vi "DbFetchRecordThroughRecordNumber.vi"() -> ()   [LabVIEW 2019]
uses:
  <vilib>/addons/database/Recordset.llb/Rec Properties.ctl
  <vilib>/addons/database/Auxilliary.llb/DB Tools Cursor Type.ctl
  <vilib>/addons/database/Connection.llb/DB Tools Open Connec (String).vi
  <vilib>/addons/database/Connection.llb/Conn Execute.vi
  <vilib>/addons/database/Recordset.llb/Rec Get Recordset Properties (R).vi
  <vilib>/addons/database/Recordset.llb/Rec Move To Record N (R).vi
  <vilib>/addons/database/Recordset.llb/Rec Fetch String Data (R).vi
  <vilib>/addons/database/Recordset.llb/Rec Destroy - Connection.vi
  <vilib>/addons/database/NI_Database_API.lvlib
panel:
  out "Subject Name":string
  in  "Provide Index of Record":dbl
  in  "stop":bool
  in  "Get Records":bool
  out "Recordset Properties":T1
  in  "Table Name":string
  in  "Provide your ODBC server name":string
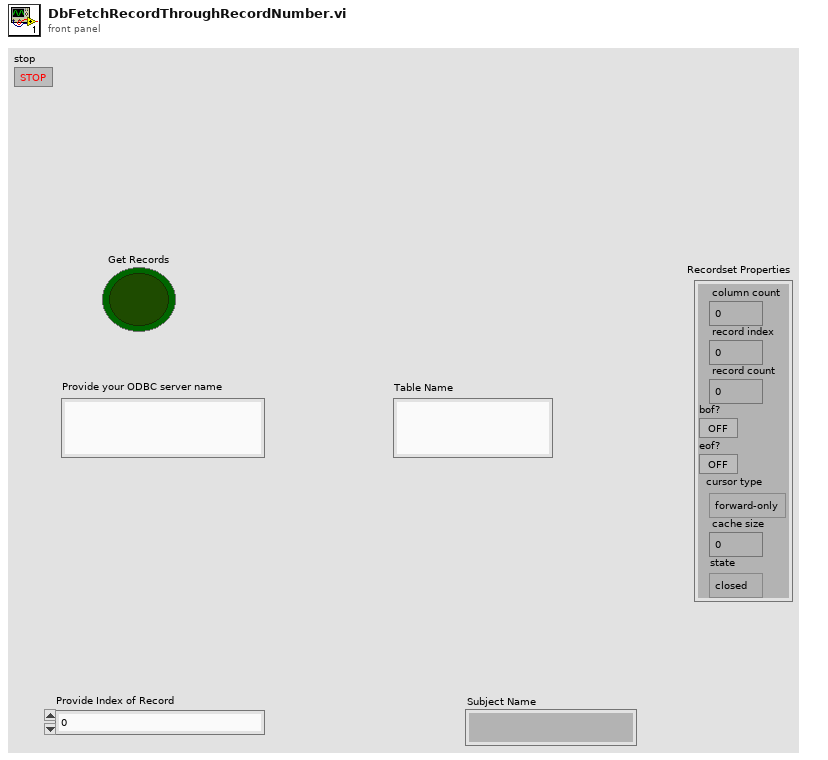
[diagram p1: front panel]
types:
  T1 = typedef "NI_Database_API.lvlib/Rec Properties.ctl" = cluster{"column count":i32, "record index":i32, "record count":i32, "bof?":bool, "eof?":bool, "cursor type":T2, "cache size":i32, "state":enum16{"closed", "open"}}
  T2 = typedef "NI_Database_API.lvlib/DB Tools Cursor Type.ctl" = enum16{"forward-only", "keyset", "dynamic", "static"}
  T3 = typedef "NI_Database_API.lvlib/Conn ObjectReference.ctl" = refnum<k1>
  T4 = typedef "NI_Database_API.lvlib/Rec ObjectReference.ctl" = refnum<k1>
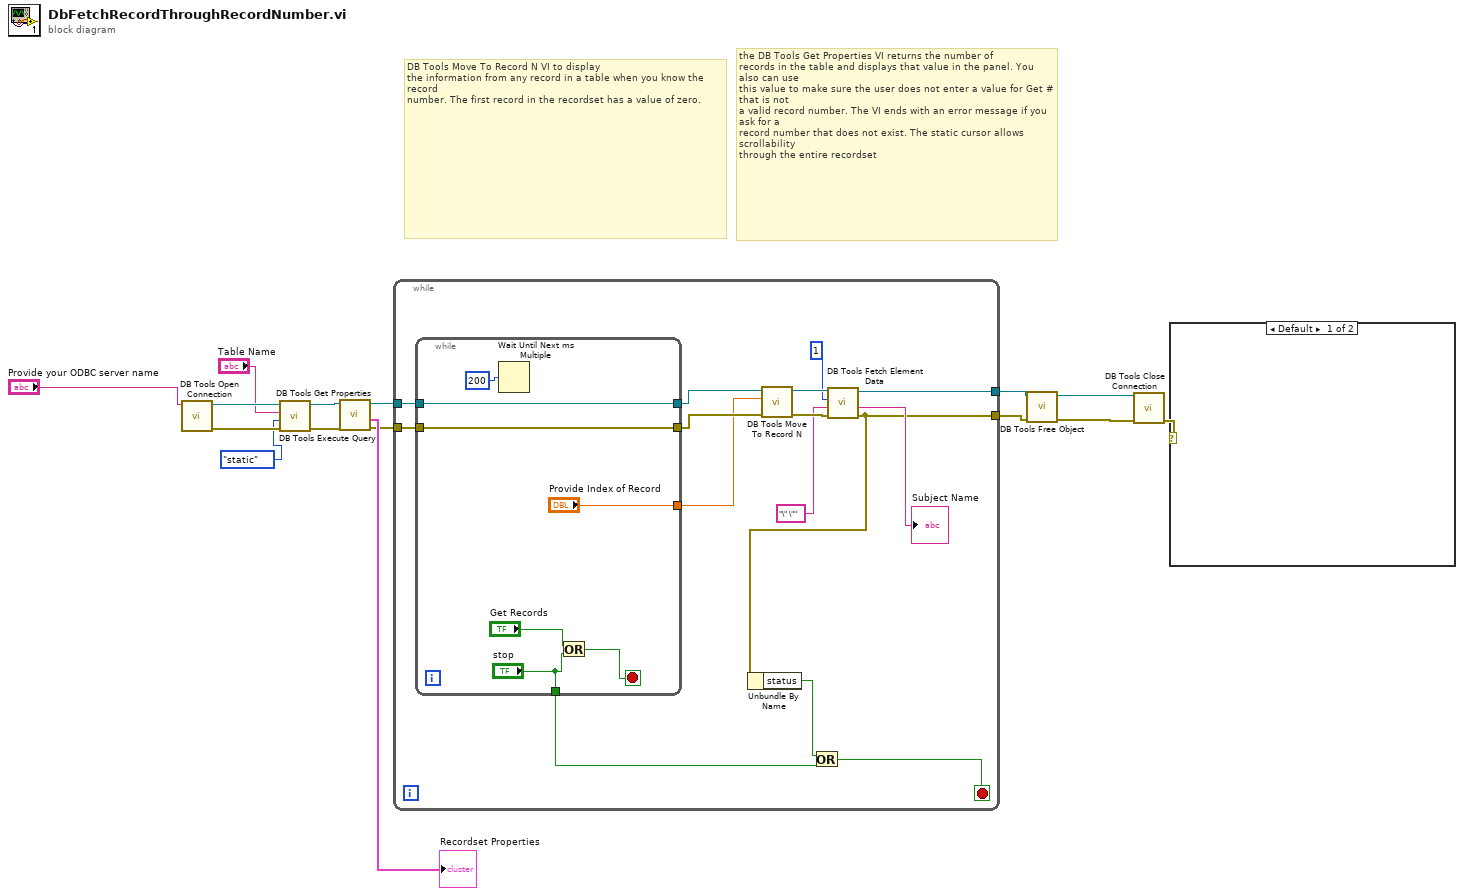
[diagram p0: block diagram]
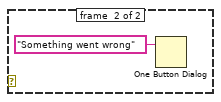
[diagram p2: hidden frame]
diagram:
  # "the DB Tools Get Properties VI returns the number of\nrecords in the table and displays that value in the panel. You also can use\nthis value to make sure the user does not enter a value for Get # that is not\na valid record number. The VI ends with an error message if you ask for a\nrecord number that does not exist. The static cursor allows scrollability\nthrough the entire recordset"
  # "DB Tools Move To Record N VI to display\nthe information from any record in a table when you know the record\nnumber. The first record in the recordset has a value of zero."
  n1 = call-poly <vilib>:"DB Tools Open Connection.vi"("connection information"="Provide your ODBC server name") -> ("error out"=w13:errorcluster, "connection reference"=w14:T3)  [unwired: 7 in]
  n2 = call-poly <vilib>:"DB Tools Execute Query.vi"("error in (no error)"=w13, "cursor type"=DB_Tools_Cursor_Type."static", "SQL query"="Table Name", "connection reference"=w14) -> ("error out"=w10:errorcluster, "recordset reference"=w9:T4)  [unwired: 4 in]
  n3 = call-poly <vilib>:"DB Tools Get Properties.vi"("error in (no error)"=w10, "recordset reference"=w9) -> ("error out"=w6:errorcluster, "recordset properties"=→"Recordset Properties":T1, "recordset reference out"=w7:T4)  [unwired: 3 in]
  n4 = while {
    tunnel: w7 -> [w30]
    tunnel: w6 -> [w29]
    tunnel: [w21] -> w5
    tunnel: [w19] -> w4
    stop <- w16 stop-if-true
    n5 = while {
      tunnel: ["Provide Index of Record"] -> w20
      tunnel: w30 -> [w33]
      tunnel: w29 -> [w32]
      tunnel: [w33] -> w28
      tunnel: [w32] -> w27
      tunnel: ["stop"] -> w18
      stop <- w36 stop-if-true
      n6 = Wait Until Next ms Multiple(millisecond multiple=u32 200) -> ()  [unwired: 1 out]
      n7 = Or(x="Get Records", y="stop") -> (x .or. y?=w36:bool)
    }
    n8 = call-poly <vilib>:"DB Tools Move To Record N.vi"("error in (no error)"=w27, "n (0)"=w20, "recordset reference"=w28) -> ("error out"=w25:errorcluster, "recordset reference out"=w26:T4)  [unwired: 7 in]
    n9 = call-poly <vilib>:"DB Tools Fetch Element Data.vi"("error in (no error)"=w25, "type"="\" \"", "column index"=1, "recordset reference"=w26) -> ("error out"=w19:errorcluster, "data"=→"Subject Name":string, "recordset reference out"=w21:T4)  [unwired: 3 in]
    n10 = Unbundle By Name(w19) -> ("status"=w17:bool)
    n11 = Or(x=w17, y=w18) -> (x .or. y?=w16:bool)
  }
  n12 = call-poly <vilib>:"DB Tools Free Object.vi"("error in (no error)"=w4, "recordset reference"=w5) -> ("error out"=w2:errorcluster, "connection reference"=w3:T3)  [unwired: 8 in]
  n13 = call <vilib>:"DB Tools Close Connection.vi"("error in (no error)"=w2, "connection reference"=w3) -> ("error out"=w1:errorcluster)  [unwired: 5 in]
  n14 = case shown="Default" w1 {
    frame #0 {
    }
    frame #1 {
      n15 = One Button Dialog(message="Something went wrong") -> ()  [unwired: 1 in, 1 out]
    }
  }
